vi "Process Data.vi"(7 "AdasLvTemplate in":refnum<class "AdasLvTemplate.lvclass">, 8 "error in":errorcluster, 11 "Node in":refnum<class "AMS Power Supply Template.lvclass">) -> (0 "error out":errorcluster, 3 "Node out":refnum<class "AMS Power Supply Template.lvclass">, 5 "AdasLvTemplate out":refnum<class "AdasLvTemplate.lvclass">)   [LabVIEW 2023, in "AMS Power Supply Template.lvlib" / "AMS Power Supply Template.lvclass"]
uses:
  AMS Power Supply Template.lvclass
  <vilib>/ADAS Replay HIL/ADAS Plugin Utilities/AdasLvTemplate/AdasLvTemplate.lvclass
  AMS Power Supply Template.lvclass/AMS Power Supply Template.ctl
  C:/Program Files/National Instruments/AMS plugin/Capabilities/Capabilities/High Level Capabilities/Power Supply Cluster/Power Supply Cluster.lvclass
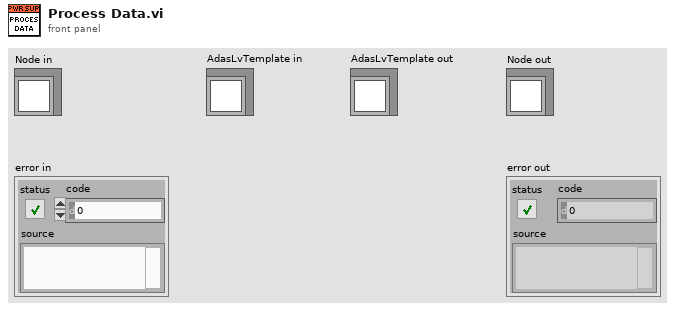
[diagram p1: front panel]
types:
  T1 = typedef "Power Supply Cluster.lvclass/Consumer Ch.ctl" = cluster{"ErrorAcknowledge.ACT":bool, "OutputEnable.ACT":bool, "ControlMode.CTL":u16, "Voltage.SP":dbl, "VoltageMIN.SP":dbl, "VoltageMAX.SP":dbl, "VoltageGrad.SP":dbl, "Current.SP":dbl, "CurrentMIN.SP":dbl, "CurrentMAX.SP":dbl, "CurrentGrad.SP":dbl, "Power.SP":dbl, "PowerMIN.SP":dbl, "PowerMAX.SP":dbl, "PowerGrad.SP":dbl}
  T2 = typedef "Power Supply Cluster.lvclass/Consumer Control.ctl" = cluster{"OnOff.ACT":bool, "ErrorAcknowledge.ACT":bool}
  T3 = typedef "Power Supply Cluster.lvclass/Producer Ch.ctl" = cluster{"Error.STS":i32, "OutputEnable.STS":i32, "ControlMode.STS":u16, "Voltage.AV":dbl, "Current.AV":dbl, "Power.AV":dbl}
  T4 = typedef "Power Supply Cluster.lvclass/Producer Control.ctl" = cluster{"OnOff.STS":i32, "Error.STS":i32, "Watchdog.STS":i32}
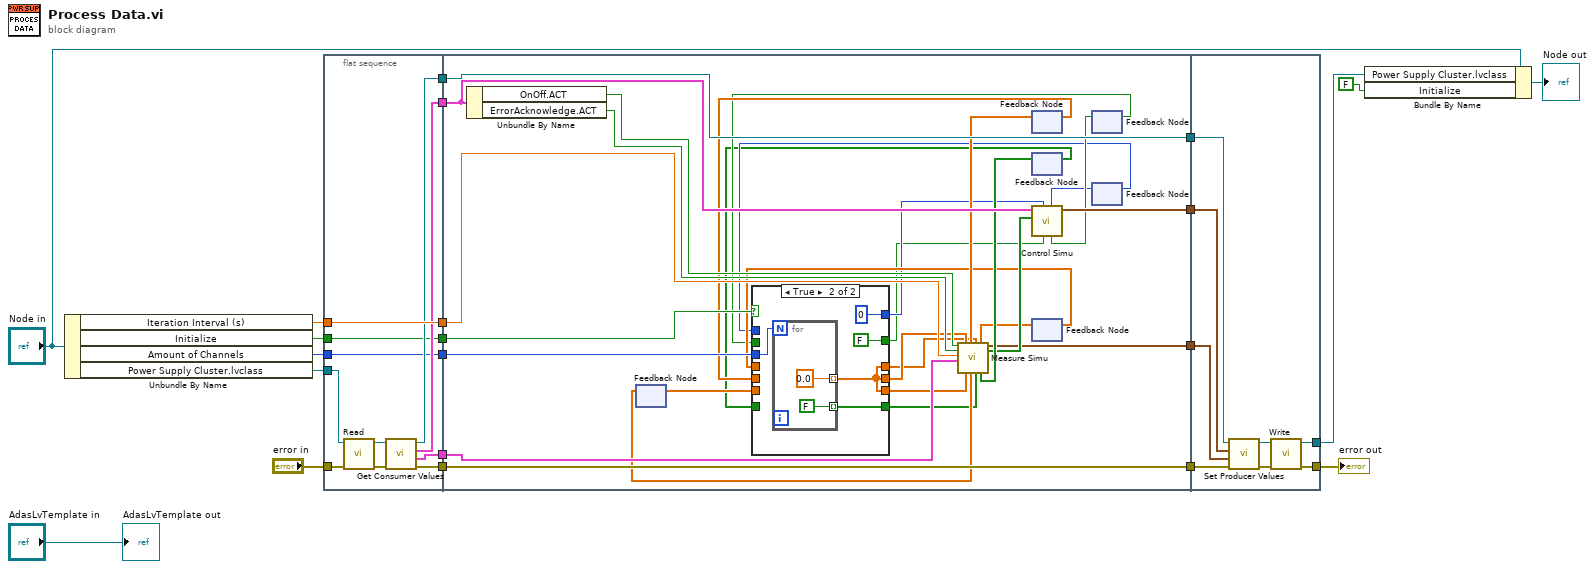
[diagram p0: block diagram]
diagram:
  n1 = Unbundle By Name("Node in") -> ("Iteration Interval (s)"=w11:dbl, "Initialize"=w4:bool, "Amount of Channels"=w3:u32, "Power Supply Cluster.lvclass"=w6:refnum<class "Power Supply Cluster.lvclass">)
  n2 = flat-sequence {
    tunnel: w6 -> [w32]
    tunnel: "error in" -> [w31]
    tunnel: [w25] -> w21
    tunnel: [w27] -> w20
    tunnel: w11 -> [w33]
    tunnel: [w33] -> w19
    tunnel: [w30] -> w18
    tunnel: [w29] -> w7
    tunnel: w4 -> [w24]
    tunnel: w3 -> [w23]
    tunnel: [w24] -> w2
    tunnel: [w23] -> w1
    tunnel: w21 -> [w63]
    tunnel: [w63] -> w17
    tunnel: [w61] -> w16
    tunnel: [w50] -> w15
    tunnel: w20 -> [w62]
    tunnel: [w62] -> w14
    tunnel: w19 -> [w55]
    tunnel: w18 -> [w60]
    tunnel: w7 -> [w54]
    tunnel: w2 -> [w47]
    tunnel: w1 -> [w46]
    tunnel: w17 -> [w78]
    tunnel: [w84] -> w12
    tunnel: w16 -> [w81]
    tunnel: w15 -> [w80]
    tunnel: w14 -> [w82]
    tunnel: [w83] -> w9
    frame #0 {
      n3 = call-dynamic "Read.vi"("error in"=w31, "Power Supply Cluster.lvclass in"=w32) -> ("error out"=w26:errorcluster, "Power Supply Cluster.lvclass out"=w28:refnum<class "Power Supply Cluster.lvclass">)  [unwired: 8 in]
      n4 = call "Get Consumer Values.vi"("error in"=w26, "Power Supply Cluster.lvclass in"=w28) -> ("error out"=w25:errorcluster, "Consumer Ch"=w29:T1[], "Consumer Control"=w30:T2, "Power Supply Cluster.lvclass out"=w27:refnum<class "Power Supply Cluster.lvclass">)  [unwired: 6 in]
    }
    frame #1 {
      n5 = Unbundle By Name(w60) -> ("OnOff.ACT"=w57:bool, "ErrorAcknowledge.ACT"=w56:bool)
      n6 = feedback #1() -> (w45:dbl[])  [unwired: 1 in]
      n7 = feedback #2() -> (w42:dbl[])  [unwired: 1 in]
      n8 = feedback #3() -> (w35:bool[])  [unwired: 1 in]
      n9 = feedback #4() -> (w43:dbl[])  [unwired: 1 in]
      n10 = feedback #5() -> (w37:bool)  [unwired: 1 in]
      n11 = feedback #6() -> (w39:i32)  [unwired: 1 in]
      n12 = case shown="True" w47 {
        tunnel: w46 -> [_ w74]
        tunnel: [w65 FALSE ("Error Feedback out")] -> w36
        tunnel: [w66 0 ("Watchdog Feedback Out")] -> w38
        tunnel: [w64 w71] -> w34
        tunnel: [w69 w70] -> w44
        tunnel: w45 -> [w69 _]
        tunnel: w43 -> [w67 _]
        tunnel: [w68 w70] -> w41
        tunnel: w42 -> [w68 _]
        tunnel: [w67 w70] -> w40
        tunnel: w39 -> [w66 _]
        tunnel: w37 -> [w65 _]
        tunnel: w35 -> [w64 _]
        frame False {
        }
        frame True {
          n13 = for {
            N: w74 -> [_]
            tunnel: [FALSE ("Feedback Out")] -> w71 mode=indexing
            tunnel: [0.0 ("Current Setpoint")] -> w70 mode=indexing
          }
        }
      }
      n14 = call "Measure Simu.vi"("OnOff.ACT"=w57, "ErrorAcknowledge.ACT"=w56, "Iteration Interval (s)"=w55, "Channels In"=w54, "Current Feedback In"=w41, "Voltage Feedback In"=w44, "Power Feedback In"=w40, "Error Feedback In"=w34) -> ("Current Feedback Out"=w49:dbl[], "Voltage Feedback Out"=w53:dbl[], "Power Feedback out"=w48:dbl[], "Error Feedback Out"=w52:bool[], "Channels Out"=w50:T3[], "Error Out"=w51:bool[])  [unwired: 6 in]
      n15 = feedback-in #1(w53) -> ()
      n16 = feedback-in #2(w49) -> ()
      n17 = feedback-in #3(w52) -> ()
      n18 = call "Control Simu.vi"("Error Feedback"=w36, "Watchdog Feedback In"=w38, "Error Ch"=w51, "Controls In"=w60) -> ("Controls Out"=w61:T4, "Error Feedback out"=w59:bool, "Watchdog Feedback Out"=w58:i32)  [unwired: 5 in]
      n19 = feedback-in #4(w48) -> ()
      n20 = feedback-in #5(w59) -> ()
      n21 = feedback-in #6(w58) -> ()
    }
    frame #2 {
      n22 = call "Set Producer Values.vi"("error in"=w78, "Producer Ch"=w80, "Producer Control"=w81, "Power Supply Cluster.lvclass in"=w82) -> ("error out"=w77:errorcluster, "Power Supply Cluster.lvclass out"=w79:refnum<class "Power Supply Cluster.lvclass">)  [unwired: 6 in]
      n23 = call-dynamic "Write.vi"("error in"=w77, "Power Supply Cluster.lvclass in"=w79) -> ("error out"=w84:errorcluster, "Power Supply Cluster.lvclass out"=w83:refnum<class "Power Supply Cluster.lvclass">)  [unwired: 8 in]
    }
  }
  n24 = Bundle By Name(cluster="Node in", "Power Supply Cluster.lvclass"=w9, "Initialize"=FALSE) -> (→"Node out":refnum<class "AMS Power Supply Template.lvclass">)
  "error out" <- w12
  "AdasLvTemplate out" <- "AdasLvTemplate in"
